vi "get_timetrace_data_from_cursors.vi"(8 "error in (no error)":errorcluster, 11 "WaveformGraph in":refnum<vi>) -> (0 "error out":errorcluster, 1 "Array 2":dbl[](array[numeric]), 2 "Array":dbl[](array[numeric]), 3 "mean":dbl)   [LabVIEW 2012]
uses:
  <vilib>/Analysis/baseanly.llb/Mean (DBL).vi
  <vilib>/Analysis/NI_AALBase.lvlib
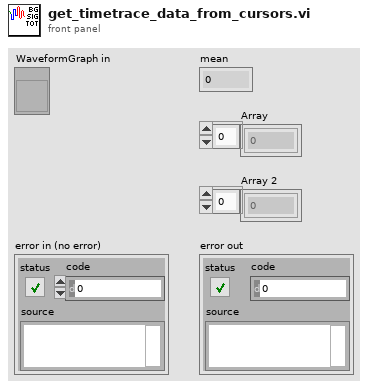
[diagram p1: front panel]
types:
  T1 = typedef "LVCursorListTypeDef.ctl" = cluster{"Name":string, "Color":u32, "Style":u8, "Point Style":u8, "Name Visible":bool, "Allow Drag":bool, "Cursor Mode":u32, "Plot":i32, "Index":i32, "Position":cluster{"X":dbl, "Y":dbl}, "X Scale":u32, "Y Scale":u32, "Watch Plots":i32[], "Watch All Plots":bool, "Plot Area":i32, "Label Offset":cluster{"X":dbl, "Y":dbl}}[]
  T2 = cluster{"CrsrList[0]":cluster{"Name":string, "Color":u32, "Style":u8, "Point Style":u8, "Name Visible":bool, "Allow Drag":bool, "Cursor Mode":u32, "Plot":i32, "Index":i32, "Position":cluster{"X":dbl, "Y":dbl}, "X Scale":u32, "Y Scale":u32, "Watch Plots":i32[], "Watch All Plots":bool, "Plot Area":i32, "Label Offset":cluster{"X":dbl, "Y":dbl}}, "CrsrList[1]":cluster{"Name":string, "Color":u32, "Style":u8, "Point Style":u8, "Name Visible":bool, "Allow Drag":bool, "Cursor Mode":u32, "Plot":i32, "Index":i32, "Position":cluster{"X":dbl, "Y":dbl}, "X Scale":u32, "Y Scale":u32, "Watch Plots":i32[], "Watch All Plots":bool, "Plot Area":i32, "Label Offset":cluster{"X":dbl, "Y":dbl}}, "CrsrList[2]":cluster{"Name":string, "Color":u32, "Style":u8, "Point Style":u8, "Name Visible":bool, "Allow Drag":bool, "Cursor Mode":u32, "Plot":i32, "Index":i32, "Position":cluster{"X":dbl, "Y":dbl}, "X Scale":u32, "Y Scale":u32, "Watch Plots":i32[], "Watch All Plots":bool, "Plot Area":i32, "Label Offset":cluster{"X":dbl, "Y":dbl}}, "CrsrList[3]":cluster{"Name":string, "Color":u32, "Style":u8, "Point Style":u8, "Name Visible":bool, "Allow Drag":bool, "Cursor Mode":u32, "Plot":i32, "Index":i32, "Position":cluster{"X":dbl, "Y":dbl}, "X Scale":u32, "Y Scale":u32, "Watch Plots":i32[], "Watch All Plots":bool, "Plot Area":i32, "Label Offset":cluster{"X":dbl, "Y":dbl}}, "CrsrList[4]":cluster{"Name":string, "Color":u32, "Style":u8, "Point Style":u8, "Name Visible":bool, "Allow Drag":bool, "Cursor Mode":u32, "Plot":i32, "Index":i32, "Position":cluster{"X":dbl, "Y":dbl}, "X Scale":u32, "Y Scale":u32, "Watch Plots":i32[], "Watch All Plots":bool, "Plot Area":i32, "Label Offset":cluster{"X":dbl, "Y":dbl}}, "CrsrList[5]":cluster{"Name":string, "Color":u32, "Style":u8, "Point Style":u8, "Name Visible":bool, "Allow Drag":bool, "Cursor Mode":u32, "Plot":i32, "Index":i32, "Position":cluster{"X":dbl, "Y":dbl}, "X Scale":u32, "Y Scale":u32, "Watch Plots":i32[], "Watch All Plots":bool, "Plot Area":i32, "Label Offset":cluster{"X":dbl, "Y":dbl}}, "CrsrList[6]":cluster{"Name":string, "Color":u32, "Style":u8, "Point Style":u8, "Name Visible":bool, "Allow Drag":bool, "Cursor Mode":u32, "Plot":i32, "Index":i32, "Position":cluster{"X":dbl, "Y":dbl}, "X Scale":u32, "Y Scale":u32, "Watch Plots":i32[], "Watch All Plots":bool, "Plot Area":i32, "Label Offset":cluster{"X":dbl, "Y":dbl}}, "CrsrList[7]":cluster{"Name":string, "Color":u32, "Style":u8, "Point Style":u8, "Name Visible":bool, "Allow Drag":bool, "Cursor Mode":u32, "Plot":i32, "Index":i32, "Position":cluster{"X":dbl, "Y":dbl}, "X Scale":u32, "Y Scale":u32, "Watch Plots":i32[], "Watch All Plots":bool, "Plot Area":i32, "Label Offset":cluster{"X":dbl, "Y":dbl}}, "CrsrList[8]":cluster{"Name":string, "Color":u32, "Style":u8, "Point Style":u8, "Name Visible":bool, "Allow Drag":bool, "Cursor Mode":u32, "Plot":i32, "Index":i32, "Position":cluster{"X":dbl, "Y":dbl}, "X Scale":u32, "Y Scale":u32, "Watch Plots":i32[], "Watch All Plots":bool, "Plot Area":i32, "Label Offset":cluster{"X":dbl, "Y":dbl}}}
  T3 = cluster{"Name":string, "Color":u32, "Style":u8, "Point Style":u8, "Name Visible":bool, "Allow Drag":bool, "Cursor Mode":u32, "Plot":i32, "Index":i32, "Position":cluster{"X":dbl, "Y":dbl}, "X Scale":u32, "Y Scale":u32, "Watch Plots":i32[], "Watch All Plots":bool, "Plot Area":i32, "Label Offset":cluster{"X":dbl, "Y":dbl}}
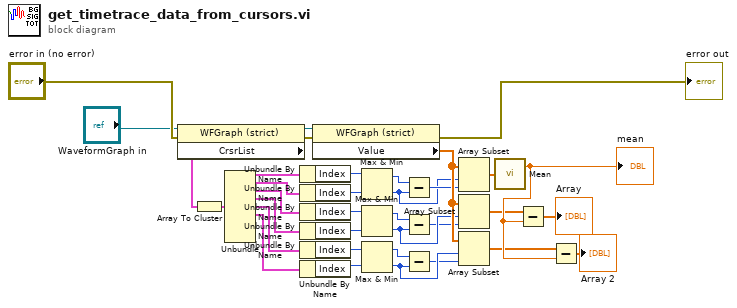
[diagram p0: block diagram]
diagram:
  n1 = property class="WFGraph (strict)"(reference="WaveformGraph in", error in="error in (no error)") -> (reference out=w17:refnum<vi>, error out=w18:errorcluster, "CrsrList"=w2:T1)
  n2 = Array To Cluster(array=w2) -> (cluster=w3:T2)
  n3 = Unbundle(w3) -> ("CrsrList[0]"=w4:T3, "CrsrList[1]"=w5:T3, "CrsrList[2]"=w6:T3, "CrsrList[3]"=w7:T3, "CrsrList[4]"=w9:T3, "CrsrList[5]"=w10:T3)  [unwired: 3 out]
  n4 = Unbundle By Name(w4) -> ("Index"=w11:i32)
  n5 = Unbundle By Name(w5) -> ("Index"=w12:i32)
  n6 = Unbundle By Name(w6) -> ("Index"=w13:i32)
  n7 = Unbundle By Name(w7) -> ("Index"=w14:i32)
  n8 = Unbundle By Name(w9) -> ("Index"=w15:i32)
  n9 = Unbundle By Name(w10) -> ("Index"=w16:i32)
  n10 = property class="WFGraph (strict)"(reference=w17, error in=w18) -> (error out=→"error out":errorcluster, "Value"=w29:dbl[])  [unwired: 1 out]
  n11 = Max & Min(x=w11, y=w12) -> (max(x,y)=w20:i32, min(x,y)=w23:i32)
  n12 = Max & Min(x=w13, y=w14) -> (max(x,y)=w21:i32, min(x,y)=w27:i32)
  n13 = Max & Min(x=w15, y=w16) -> (max(x,y)=w22:i32, min(x,y)=w28:i32)
  n14 = Subtract(x=w20, y=w23) -> (x-y=w24:i32)
  n15 = Subtract(x=w21, y=w27) -> (x-y=w25:i32)
  n16 = Subtract(x=w22, y=w28) -> (x-y=w26:i32)
  n17 = Array Subset(array=w29, index=w23, length=w24) -> (w30:dbl[])
  n18 = Array Subset(array=w29, index=w27, length=w25) -> (w33:dbl[])
  n19 = Array Subset(array=w29, index=w28, length=w26) -> (w31:dbl[])
  n20 = call-poly <vilib>:"Mean.vi"("X"=w30) -> ("mean"=w34:dbl)  [unwired: 1 out]
  "mean" <- w34
  n21 = Subtract(x=w33, y=w34) -> (x-y=→"Array":dbl[])
  n22 = Subtract(x=w31, y=w34) -> (x-y=→"Array 2":dbl[])
